vi "simple_gain_scheduler.vi"(10 "Scheduled Variable":dbl, 11 "gain_scheduler":T2) -> (3 "Gain":T1)   [LabVIEW 2011]
uses:
  gain_sched_const.ctl
  gain_const.ctl
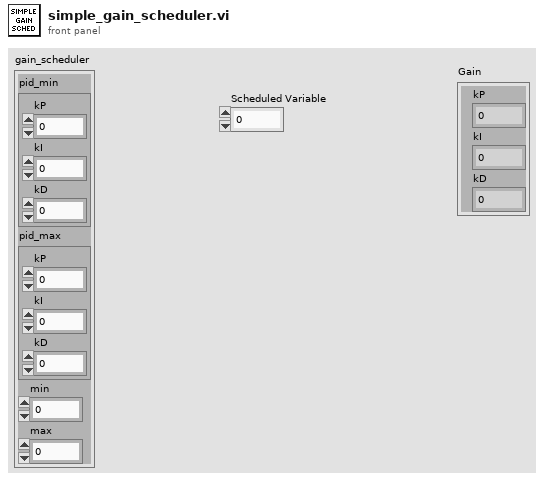
[diagram p1: front panel]
types:
  T1 = typedef "gain_const.ctl" = cluster{"kP":dbl, "kI":dbl, "kD":dbl}
  T2 = typedef "gain_sched_const.ctl" = cluster{"pid_min":T1, "pid_max":T1, "min":dbl, "max":dbl}
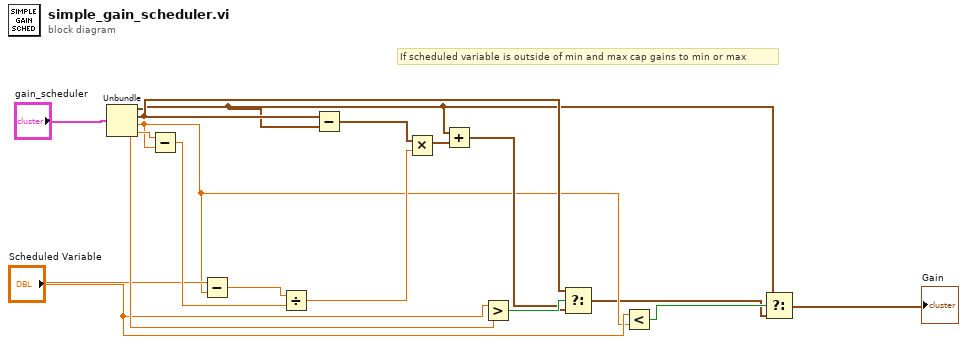
[diagram p0: block diagram]
diagram:
  # "If scheduled variable is outside of min and max cap gains to min or max"
  n1 = Unbundle("gain_scheduler") -> ("pid_min"=w2:T1, "pid_max"=w7:T1, "min"=w5:dbl, "max"=w10:dbl)
  n2 = Subtract(x=w10, y=w5) -> (x-y=w14:dbl)
  n3 = Subtract(x="Scheduled Variable", y=w5) -> (x-y=w15:dbl)
  n4 = Divide(x=w15, y=w14) -> (x/y=w12:dbl)
  n5 = Subtract(x=w7, y=w2) -> (x-y=w13:T1)
  n6 = Multiply(x=w13, y=w12) -> (x*y=w11:T1)
  n7 = Add(x=w2, y=w11) -> (x+y=w8:T1)
  n8 = Greater?(x="Scheduled Variable", y=w10) -> (0:w9:bool)
  n9 = Select(t=w7, s=w9, f=w8) -> (s? t:f=w3:T1)
  n10 = Less?(x="Scheduled Variable", y=w5) -> (x < y?=w4:bool)
  n11 = Select(t=w2, s=w4, f=w3) -> (s? t:f=→"Gain":T1)
